vi "Msg.vi"(7 "jettl in":refnum<class "jettl.lvclass">, 11 "Override Error Msg Strategy in":refnum<class "Override Error Msg Strategy.lvclass">) -> (5 "jettl out":refnum<class "jettl.lvclass">)   [LabVIEW 2021, in "jettl Msg Override Error.lvlib" / "Override Error Msg Strategy.lvclass"]
uses:
  Override Error Msg Strategy.lvclass
  jettl/jettl/jettl.lvclass
  jettl Msg Override Error/jettl Msg Override Error.lvclass
  Override Error Msg Strategy.lvclass/Override Error Msg Strategy.ctl
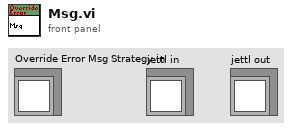
[diagram p1: front panel]
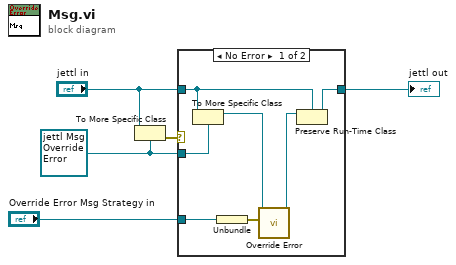
[diagram p0: block diagram]
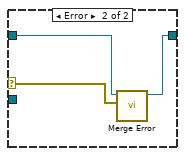
[diagram p2: hidden frame]
diagram:
  w2 = refnum<class "jettl Msg Override Error.lvclass"> refnum ("jettl.lvlib:Override Error.lvlib:Override Error.lvclass")
  n1 = To More Specific Class(target class=w2, reference="jettl in") -> (error out=w5:errorcluster)  [unwired: 1 in, 1 out]
  n2 = case shown="No Error" w5 {
    selector: w5 -> [_ w15]
    tunnel: [w10 w13] -> w1
    tunnel: "jettl in" -> [w11 w14]
    tunnel: w2 -> [w12 _]
    tunnel: "Override Error Msg Strategy in" -> [w7 _]
    frame No Error {
      n3 = To More Specific Class(target class=w12, reference=w11) -> (specific class reference=w8:refnum<class "jettl Msg Override Error.lvclass">)  [unwired: 1 in, 1 out]
      n4 = Unbundle(w7) -> (w6:errorcluster)
      n5 = call-dynamic "Override Error.vi"("Error"=w6, "jettl Msg Override Error in"=w8) -> ("jettl Msg Override Error out"=w9:refnum<class "jettl Msg Override Error.lvclass">)  [unwired: 9 in]
      n6 = Preserve Run-Time Class(object in=w9, 2:w11) -> (object out=w10:refnum<class "jettl.lvclass">)  [unwired: 1 in, 1 out]
    }
    frame Error {
      n7 = call-dynamic "Merge Error.vi"("Error"=w15, "jettl Msg Merge Error in"=w14) -> ("jettl Msg Merge Error out"=w13:refnum<class "jettl.lvclass">)  [unwired: 9 in]
    }
  }
  "jettl out" <- w1
